vi "Set Data.vi"(8 "error in (no error)":errorcluster, 10 "Data":refnum<class "Data.lvclass">, 11 "Signal in":refnum<class "Signal.lvclass">) -> (0 "error out":errorcluster, 3 "Signal out":refnum<class "Signal.lvclass">)   [LabVIEW 2015, in "MDSplus.lvlib" / "Signal.lvclass"]
uses:
  <vilib>/MDSplus/Classes/Data_Class/Compound_Class/Signal_Class/Signal.lvclass
  <vilib>/MDSplus/Classes/Data_Class/Data.lvclass
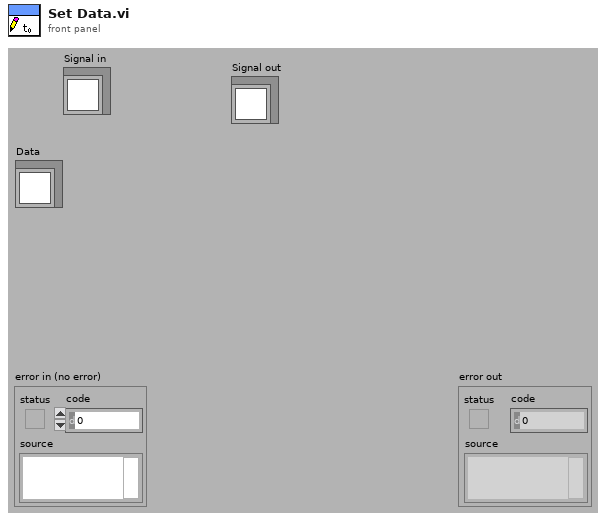
[diagram p1: front panel]
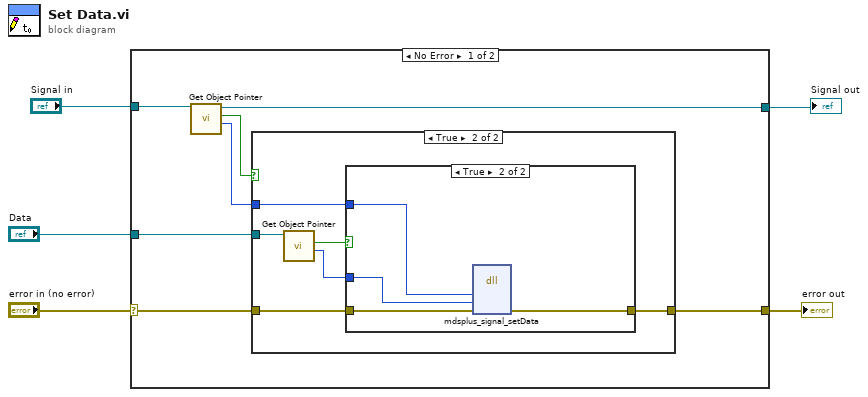
[diagram p0: block diagram]
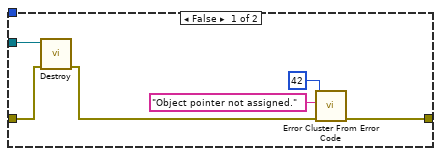
[diagram p2: hidden frame]
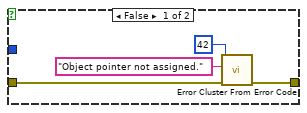
[diagram p3: hidden frame]
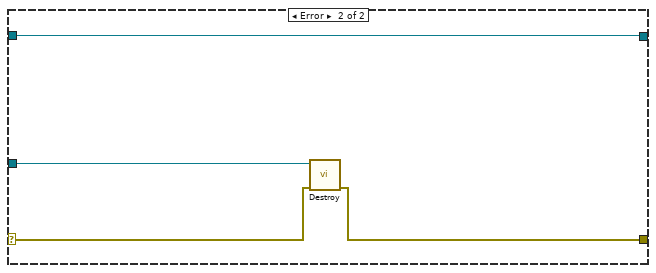
[diagram p4: hidden frame]
diagram:
  n1 = case shown="No Error" "error in (no error)" {
    selector: "error in (no error)" -> [w9 w35]
    tunnel: [w8 w34] -> w4
    tunnel: [w7 w33] -> w1
    tunnel: "Data" -> [w12 w36]
    tunnel: "Signal in" -> [w6 w33]
    frame No Error {
      n2 = call-dynamic "Get Object Pointer.vi"("Data in"=w6) -> ("Object Pointer"=w10:i64, "Assigned object pointer?"=w11:bool, "Data out"=w7:refnum<class "Signal.lvclass">)  [unwired: 8 in]
      n3 = case shown="True" w11 {
        tunnel: w12 -> [w15 w24]
        tunnel: w10 -> [_ w21]
        tunnel: w9 -> [w14 w20]
        tunnel: [w16 w19] -> w8
        frame False {
          n4 = call-dynamic "Destroy.vi"("error in (no error)"=w14, "Data in"=w15) -> ("error out"=w13:errorcluster)  [unwired: 9 in]
          n5 = call <vilib>:"Error Cluster From Error Code.vi"("error in (no error)"=w13, "error message (\"\")"="Object pointer not assigned." ("error message (\"\")"), "error code (0)"=42) -> ("error out"=w16:errorcluster)  [unwired: 6 in]
        }
        frame True {
          n6 = call-dynamic "Get Object Pointer.vi"("Data in"=w24) -> ("Object Pointer"=w22:i64, "Assigned object pointer?"=w23:bool)  [unwired: 8 in, 1 out]
          n7 = case shown="True" w23 {
            tunnel: w22 -> [_ w31]
            tunnel: w21 -> [_ w32]
            tunnel: w20 -> [w26 w30]
            tunnel: [w25 w29] -> w19
            frame False {
              n8 = call <vilib>:"Error Cluster From Error Code.vi"("error in (no error)"=w26, "error message (\"\")"="Object pointer not assigned." ("error message (\"\")"), "error code (0)"=42) -> ("error out"=w25:errorcluster)  [unwired: 6 in]
            }
            frame True {
              n9 = dll-call lib="MDSobjectsLVShr" fn="mdsplus_signal_setData"("lvSignalPtr"=w32, "lvDataPtrIn"=w31, "error"=w30) -> ("error"=w29:errorcluster)  [unwired: 6 in, 2 out]
            }
          }
        }
      }
    }
    frame Error {
      n10 = call-dynamic "Destroy.vi"("error in (no error)"=w35, "Data in"=w36) -> ("error out"=w34:errorcluster)  [unwired: 9 in]
    }
  }
  "error out" <- w4
  "Signal out" <- w1
